vi "OperationCall.vi"(0 "Subtract in":refnum<class "Subtract.lvclass">, 5 "Sub Panel":refnum<vi>, 7 "user event out":refnum<user-event>, 9 "event source":refnum<user-event>, 11 "error in (no error)":errorcluster) -> (4 "Subtract out":refnum<class "Subtract.lvclass">, 15 "error out":errorcluster)   [LabVIEW 2023, in "Subtract.lvclass"]
uses:
  Subtract.lvclass
  Arithmetic/Arithmetic.lvclass
  SubtractionUI.vi
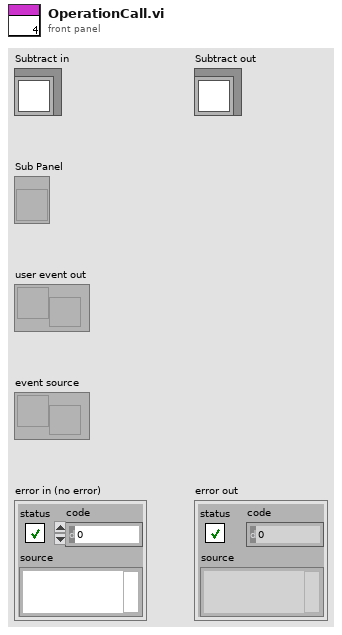
[diagram p1: front panel]
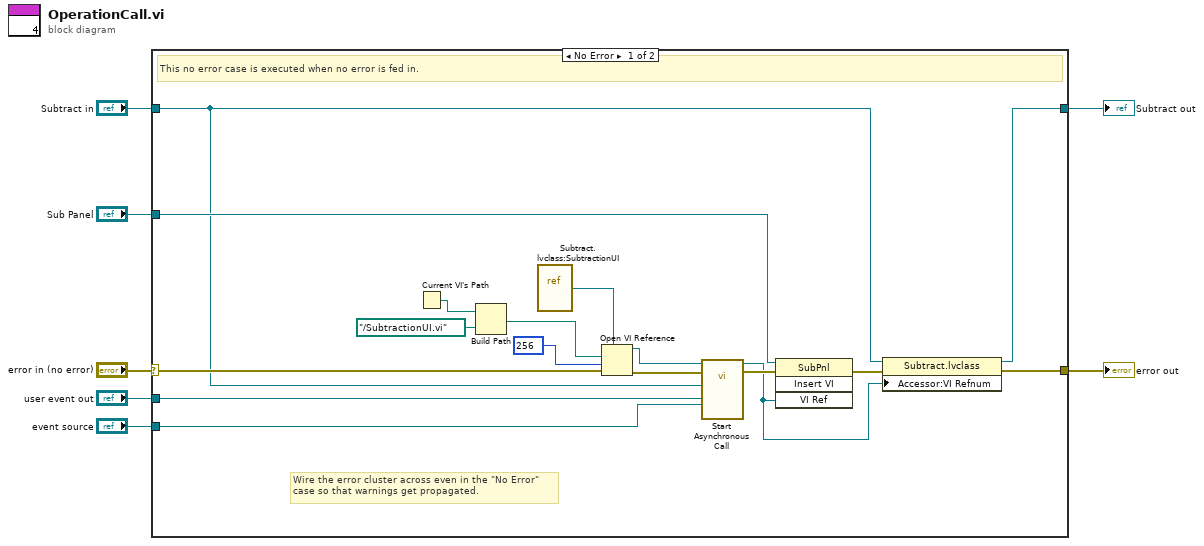
[diagram p0: block diagram]
diagram:
  n1 = case shown="No Error" "error in (no error)" {
    selector: "error in (no error)" -> [w12 w26]
    tunnel: [w13 w26] -> w6
    tunnel: [w10 w25] -> w4
    tunnel: "Subtract in" -> [w8 w25]
    tunnel: "user event out" -> [w17 _]
    tunnel: "event source" -> [w14 _]
    tunnel: "Sub Panel" -> [w16 _]
    frame No Error {
      # "Wire the error cluster across even in the \"No Error\"\ncase so that warnings get propagated."
      # "This no error case is executed when no error is fed in."
      n2 = Current VI's Path() -> (path=w15:path)
      n3 = Build Path(base path=w15, name or relative path=path "../SubtractionUI.vi") -> (appended path=w20:path)
      n4 = vi-ref "Subtract.lvclass:SubtractionUI.vi"() -> (w23:refnum<vi>)
      n5 = Open VI Reference(type specifier VI Refnum (for type only)=w23, vi path=w20, options=256, error in (no error)=w12) -> (vi reference=w18:refnum<vi>, error out=w21:errorcluster)  [unwired: 2 in]
      n6 = call-by-ref "Start Asynchronous Call"(reference=w18, error in=w21, "Subtract in"=w8, "user event out"=w17, "event source"=w14) -> (reference out=w9:refnum<vi>, error out=w22:errorcluster)  [unwired: 10 in, 3 out]
      n7 = invoke on="Invoke Node" class="SubPnl" method="Insert VI"(reference=w16, error in=w22, "VI Ref"=w9) -> (error out=w11:errorcluster)  [unwired: 1 in, 3 out]
      n8 = property class="Subtract.lvclass"(reference=w8, error in=w11, "Accessor:VI Refnum"=w9) -> (reference out=w10:refnum<class "Subtract.lvclass">, error out=w13:errorcluster)
    }
    frame Error {
      # "This error case is executed when error is fed in and fed out through error out."
    }
  }
  "error out" <- w6
  "Subtract out" <- w4
